vi "GSP_arraytosrting.vi"(0 "Array In":string[](array[string]), 1 "char between elements":string) -> (5 "String out":string)   [LabVIEW 2015]
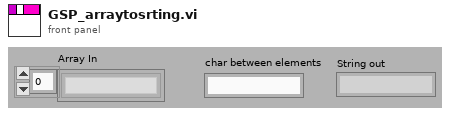
[diagram p1: front panel]
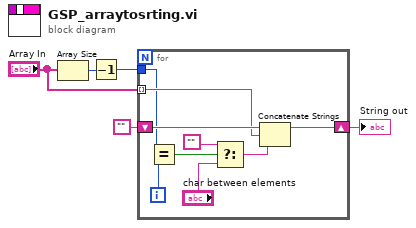
[diagram p0: block diagram]
diagram:
  n1 = Array Size(array="Array In") -> (size(s)=w4:i32)
  n2 = Decrement(x=w4) -> (x-1=w1:i32)
  n3 = for {
    shift-right: [w14] -> w2
    shift-left: "" -> [w13]
    tunnel: "Array In" -> [w12] mode=indexing
    tunnel: w1 -> [w6]
    i -> [w9]
    n4 = Equal?(x=w6, y=w9) -> (x = y?=w8:bool)
    n5 = Select(t="", s=w8, f="char between elements") -> (s? t:f=w11:string)
    n6 = Concatenate Strings(w13, w12, w11) -> (w14:string)
  }
  "String out" <- w2
